vi "Set Advanced Triggering Mode.vi"(8 "error in (no error)":errorcluster, 10 "Enable Adv Trig Mode":bool, 11 "VISA resource name":refnum<visa-resource-name>) -> (0 "error out":errorcluster, 3 "VISA resource name out":refnum<visa-resource-name>, 4 "Device Errors":cluster{"code":i32, "Text":string}[](array[cluster]))   [LabVIEW 2014, in "Stanford Research DG645 - Driver.lvlib"]
doc: "Trigger Command: ADVT i\nInstrument Error Check\n\nSet the advanced triggering enable register to i. If i is false (0), advanced triggering is disabled. If i is true (1), advanced triggering is enabled."
uses:
  Stanford Research DG645 - Driver.lvlib
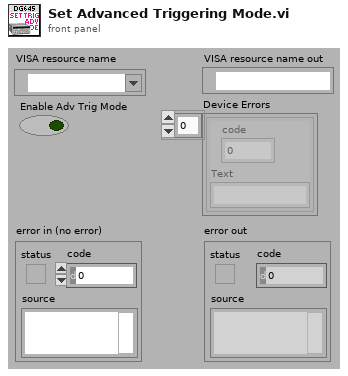
[diagram p1: front panel]
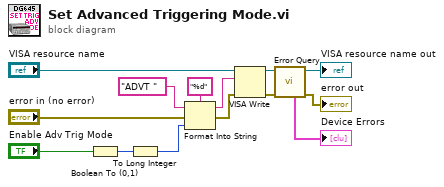
[diagram p0: block diagram]
diagram:
  n1 = Boolean To (0,1)(Boolean="Enable Adv Trig Mode") -> (0, 1=w2:i16)
  n2 = To Long Integer(number=w2) -> (32bit integer=w1:i32)
  n3 = Format Into String(format string="%d", initial string="ADVT " ("command"), error in="error in (no error)", w1) -> (resulting string=w4:string, error out=w3:errorcluster)
  n4 = VISA Write(VISA resource name="VISA resource name", write buffer=w4, error in (no error)=w3) -> (VISA resource name out=w10:refnum<visa-resource-name>, error out=w7:errorcluster)  [unwired: 1 out]
  n5 = call "Error Query.vi"("error in (no error)"=w7, "VISA resource name"=w10) -> ("error out"=→"error out":errorcluster, "VISA resource name out"=→"VISA resource name out":refnum<visa-resource-name>, "Device Errors"=→"Device Errors":cluster{"code":i32, "Text":string}[])  [unwired: 7 in]
